vi "random.vi"   [LabVIEW 2017]
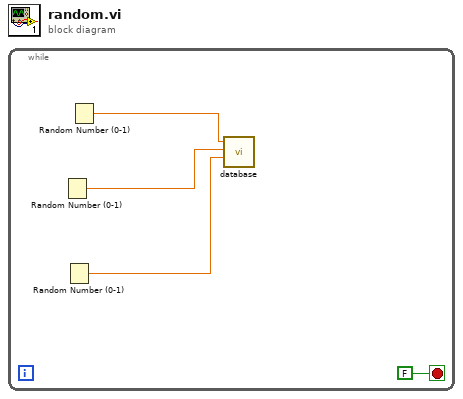
[diagram p0: block diagram]
diagram:
  n1 = while {
    stop <- FALSE stop-if-true
    n2 = Random Number (0-1)() -> (number: 0 to 1=w3:dbl)
    n3 = Random Number (0-1)() -> (number: 0 to 1=w2:dbl)
    n4 = Random Number (0-1)() -> (number: 0 to 1=w4:dbl)
    n5 = call "database.vi"("Fail_db"=w2, "Pass_db"=w3, "Total_db"=w4) -> ()  [unwired: 9 in]
  }
